vi "Create Icon String.vi"(11 "Simple Class Name":string) -> (3 "Abbriviated Icon Name":string)   [LabVIEW 2015, in "QControl Creation Wizard.lvclass"]
doc: "<b> </b> <b> </b>\n©2016 Q Software Innovations, LLC (QSI)\nwritten by Quentin Alldredge\nproduced in LabVIEW 2015\n\nsupport@qsoftwareinnovations.com\nwww.qsoftwareinnovations.com\n\nAll rights reserved.\n\nRedistribution and use in source and binary forms, with or without modification, are permitted provided that the following conditions are met:\n\n * Redistributions of source code must retain the above copyright notice, this list of conditions and the following disclaimer.\n * Redistributions in binary form must reproduce the above copyright notice, this list of conditions and the following disclaimer in the documentation and/or other materials provided with the distribution.\n * Neither the name of Q Software Innovations, LLC. nor the names of its contributors may be used to endorse or promote products derived from this software without specific prior written permission.\n\nTHIS SOFTWARE IS PROVIDED BY THE COPYRIGHT HOLDERS AND CONTRIBUTORS \"AS IS\" AND ANY EXPRESS OR IMPLIED WARRANTIES, INCLUDING, BUT NOT LIMITED TO, THE IMPLIED WARRANTIES OF MERCHANTABILITY AND FITNESS FOR A PARTICULAR PURPOSE ARE DISCLAIMED. IN NO EVENT SHALL THE COPYRIGHT OWNER OR CONTRIBUTORS BE LIABLE FOR ANY DIRECT, INDIRECT, INCIDENTAL, SPECIAL, EXEMPLARY, OR CONSEQUENTIAL DAMAGES (INCLUDING, BUT NOT LIMITED TO, PROCUREMENT OF SUBSTITUTE GOODS OR SERVICES; LOSS OF USE, DATA, OR PROFITS; OR BUSINESS INTERRUPTION) HOWEVER CAUSED AND ON ANY THEORY OF LIABILITY, WHETHER IN CONTRACT, STRICT LIABILITY, OR TORT (INCLUDING NEGLIGENCE OR OTHERWISE) ARISING IN ANY WAY OUT OF THE USE OF THIS SOFTWARE, EVEN IF ADVISED OF THE POSSIBILITY OF SUCH DAMAGE."
uses:
  QControl Creation Wizard.lvclass
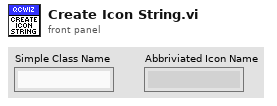
[diagram p1: front panel]
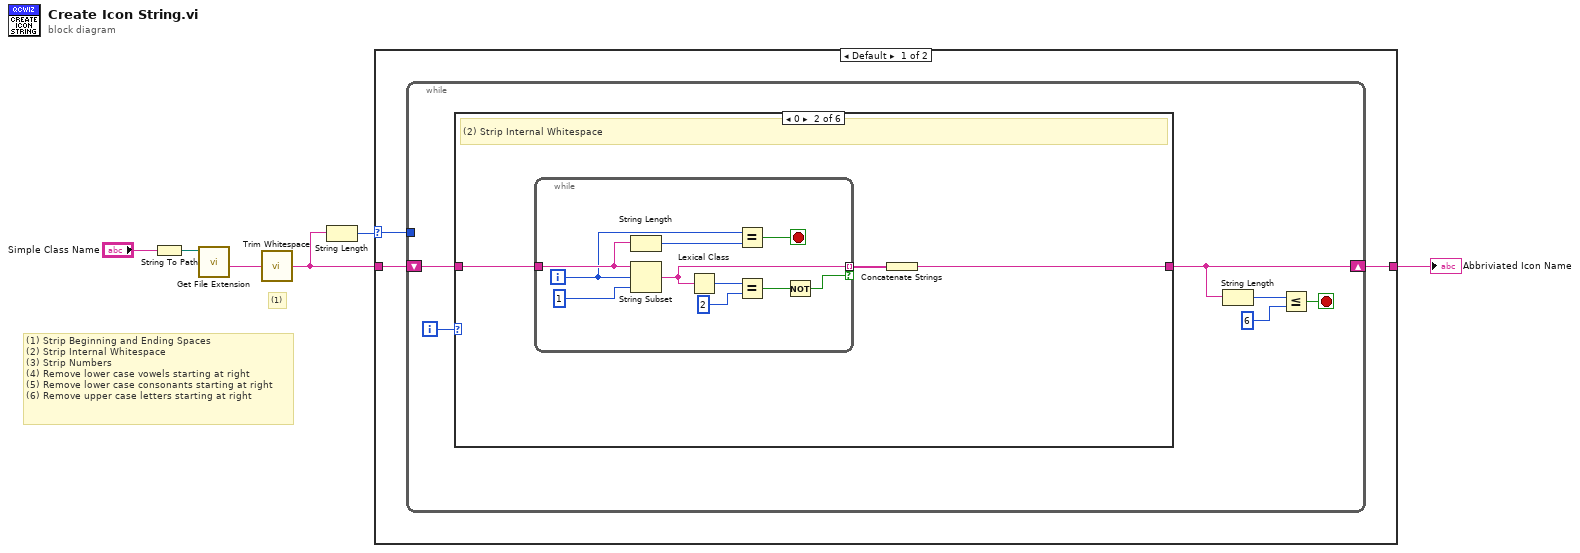
[diagram p0: block diagram]
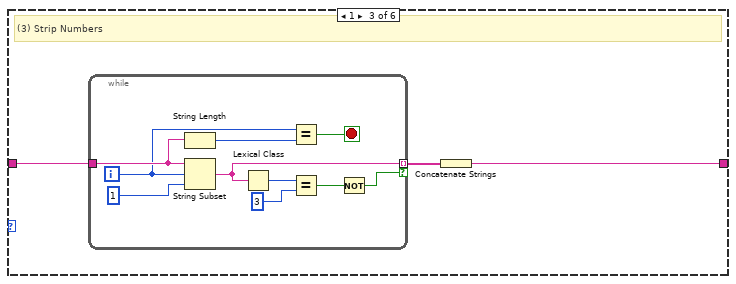
[diagram p3: hidden frame]
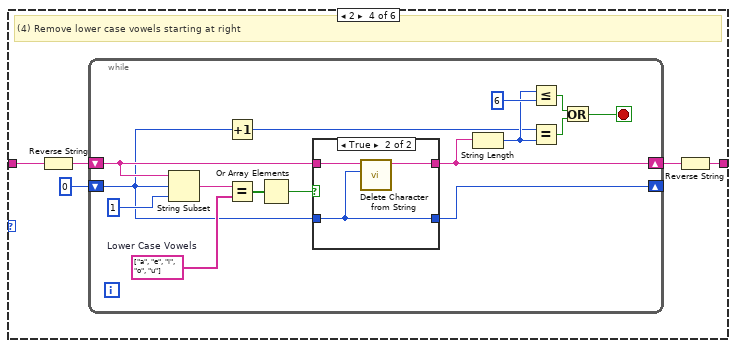
[diagram p4: hidden frame]
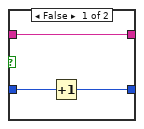
[diagram p5: hidden frame]
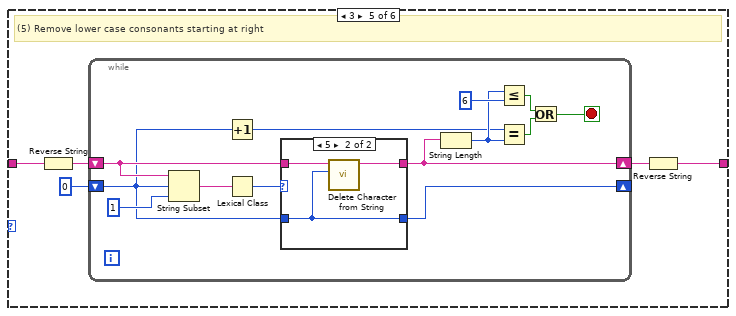
[diagram p6: hidden frame]
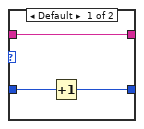
[diagram p7: hidden frame]
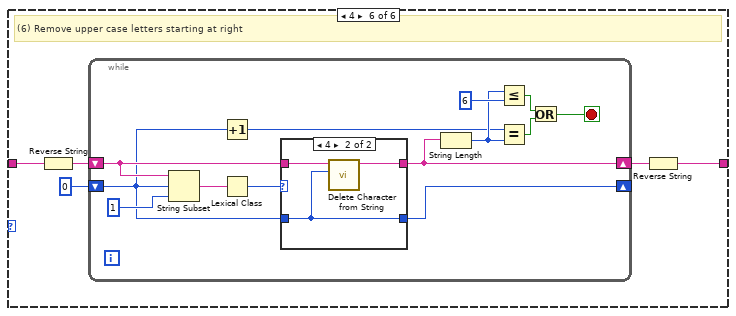
[diagram p8: hidden frame]
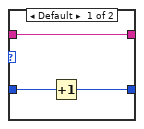
[diagram p9: hidden frame]
diagram:
  # "(1)"
  # "(1) Strip Beginning and Ending Spaces\n(2) Strip Internal Whitespace\n(3) Strip Numbers\n(4) Remove lower case vowels starting at right \n(5) Remove lower case consonants starting at right\n(6) Remove upper case letters starting at right"
  n1 = String To Path(string="Simple Class Name") -> (path=w3:path)
  n2 = call <vilib>:"Get File Extension.vi"("file"=w3) -> ("filename without extension"=w5:string)  [unwired: 6 in, 4 out]
  n3 = call <vilib>:"Trim Whitespace.vi"("string"=w5) -> ("trimmed string"=w1:string)  [unwired: 1 in]
  n4 = String Length(string=w1) -> (length=w4:i32)
  n5 = case shown="Default" w4 {
    selector: w4 -> [w7 _]
    tunnel: [w8 w117] -> w6
    tunnel: w1 -> [w9 w117]
    frame Default {
      n6 = while {
        shift-right: [w13] -> w8
        shift-left: w9 -> [w14]
        tunnel: w7 -> [_]
        i -> [w15]
        stop <- w10 stop-if-true
        n7 = case shown="0" w15 {
          tunnel: w14 -> [w16 w19 w32 w47 w73 w97]
          tunnel: [w16 w17 w30 w44 w70 w94] -> w13
          frame Default {
          }
          frame 0 {
            # "(2) Strip Internal Whitespace"
            n8 = while {
              tunnel: w19 -> [w25]
              tunnel: [w26] -> w18 mode=indexing if=w21
              i -> [w23]
              stop <- w20 stop-if-true
              n9 = String Length(string=w25) -> (length=w24:i32)
              n10 = String Subset(string=w25, offset (0)=w23, length (rest)=1 ("length (rest)")) -> (substring=w26:string)
              n11 = Lexical Class(1:w26) -> (0:w28:i16)
              n12 = Equal?(x=w23, y=w24) -> (x = y?=w20:bool)
              n13 = Equal?(x=w28, y=i16 2) -> (x = y?=w22:bool)
              n14 = Not(x=w22) -> (.not. x?=w21:bool)
            }
            n15 = Concatenate Strings(w18) -> (w17:string)
          }
          frame 1 {
            # "(3) Strip Numbers"
            n16 = while {
              tunnel: w32 -> [w38]
              tunnel: [w39] -> w31 mode=indexing if=w34
              i -> [w36]
              stop <- w33 stop-if-true
              n17 = String Length(string=w38) -> (length=w37:i32)
              n18 = String Subset(string=w38, offset (0)=w36, length (rest)=1 ("length (rest)")) -> (substring=w39:string)
              n19 = Lexical Class(1:w39) -> (0:w41:i16)
              n20 = Equal?(x=w36, y=w37) -> (x = y?=w33:bool)
              n21 = Equal?(x=w41, y=i16 3) -> (x = y?=w35:bool)
              n22 = Not(x=w35) -> (.not. x?=w34:bool)
            }
            n23 = Concatenate Strings(w31) -> (w30:string)
          }
          frame 2 {
            # "(4) Remove lower case vowels starting at right"
            n24 = Reverse String(1:w47) -> (0:w45:string)
            n25 = while {
              shift-right: [w54] -> w46
              shift-left: w45 -> [w58]
              shift-right: [w48] -> _
              shift-left: 0 -> [w49]
              stop <- w55 stop-if-true
              w60 = string[] ["a", "e", "i", "o", "u"]  # Lower Case Vowels
              n26 = String Subset(string=w58, offset (0)=w49, length (rest)=1 ("length (rest)")) -> (substring=w61:string)
              n27 = Increment(x=w49) -> (x+1=w50:i32)
              n28 = Equal?(x=w61, y=w60) -> (x = y?=w59:bool[])
              n29 = Or Array Elements(Boolean array=w59) -> (logical OR=w57:bool)
              n30 = case shown="True" w57 {
                tunnel: w58 -> [w65 w68]
                tunnel: w49 -> [w64 w66]
                tunnel: [w65 w67] -> w54
                tunnel: [w63 w66] -> w48
                frame False {
                  n31 = Increment(x=w64) -> (x+1=w63:i32)
                }
                frame True {
                  n32 = call "Delete Character from String.vi"("Index to Delete"=w66, "String in"=w68) -> ("String out"=w67:string)  [unwired: 9 in]
                }
              }
              n33 = String Length(string=w54) -> (length=w52:i32)
              n34 = Less Or Equal?(x=w52, y=6) -> (x <= y?=w51:bool)
              n35 = Equal?(x=w50, y=w52) -> (x = y?=w56:bool)
              n36 = Or(x=w51, y=w56) -> (x .or. y?=w55:bool)
            }
            n37 = Reverse String(1:w46) -> (0:w44:string)
          }
          frame 3 {
            # "(5) Remove lower case consonants starting at right"
            n38 = Reverse String(1:w73) -> (0:w71:string)
            n39 = while {
              shift-right: [w82] -> w72
              shift-left: w71 -> [w85]
              shift-right: [w74] -> _
              shift-left: 0 ("length (rest)") -> [w75]
              stop <- w83 stop-if-true
              n40 = String Subset(string=w85, offset (0)=w75, length (rest)=1 ("length (rest)")) -> (substring=w78:string)
              n41 = Increment(x=w75) -> (x+1=w76:i32)
              n42 = Lexical Class(1:w78) -> (0:w77:i16)
              n43 = case shown="5" w77 {
                tunnel: w85 -> [w89 w92]
                tunnel: w75 -> [w88 w90]
                tunnel: [w89 w91] -> w82
                tunnel: [w87 w90] -> w74
                frame Default {
                  n44 = Increment(x=w88) -> (x+1=w87:i32)
                }
                frame 5 {
                  n45 = call "Delete Character from String.vi"("Index to Delete"=w90, "String in"=w92) -> ("String out"=w91:string)  [unwired: 9 in]
                }
              }
              n46 = String Length(string=w82) -> (length=w80:i32)
              n47 = Less Or Equal?(x=w80, y=6) -> (x <= y?=w79:bool)
              n48 = Equal?(x=w76, y=w80) -> (x = y?=w84:bool)
              n49 = Or(x=w79, y=w84) -> (x .or. y?=w83:bool)
            }
            n50 = Reverse String(1:w72) -> (0:w70:string)
          }
          frame 4 {
            # "(6) Remove upper case letters starting at right"
            n51 = Reverse String(1:w97) -> (0:w95:string)
            n52 = while {
              shift-right: [w106] -> w96
              shift-left: w95 -> [w109]
              shift-right: [w98] -> _
              shift-left: 0 ("length (rest)") -> [w99]
              stop <- w107 stop-if-true
              n53 = String Subset(string=w109, offset (0)=w99, length (rest)=1 ("length (rest)")) -> (substring=w102:string)
              n54 = Increment(x=w99) -> (x+1=w100:i32)
              n55 = Lexical Class(1:w102) -> (0:w101:i16)
              n56 = case shown="4" w101 {
                tunnel: w109 -> [w113 w116]
                tunnel: w99 -> [w112 w114]
                tunnel: [w113 w115] -> w106
                tunnel: [w111 w114] -> w98
                frame Default {
                  n57 = Increment(x=w112) -> (x+1=w111:i32)
                }
                frame 4 {
                  n58 = call "Delete Character from String.vi"("Index to Delete"=w114, "String in"=w116) -> ("String out"=w115:string)  [unwired: 9 in]
                }
              }
              n59 = String Length(string=w106) -> (length=w104:i32)
              n60 = Less Or Equal?(x=w104, y=6) -> (x <= y?=w103:bool)
              n61 = Equal?(x=w100, y=w104) -> (x = y?=w108:bool)
              n62 = Or(x=w103, y=w108) -> (x .or. y?=w107:bool)
            }
            n63 = Reverse String(1:w96) -> (0:w94:string)
          }
        }
        n64 = String Length(string=w13) -> (length=w11:i32)
        n65 = Less Or Equal?(x=w11, y=6) -> (x <= y?=w10:bool)
      }
    }
    frame ..6 {
    }
  }
  "Abbriviated Icon Name" <- w6
